vi "solar Unpack.vi"(6 "Timed Out?":bool, 8 "error in (no error)":errorcluster, 9 "DATA in":variant, 10 "MSG in":string, 11 "solar in":refnum<class "solar.lvclass">) -> (0 "error out":errorcluster, 1 "DATA out":variant, 2 "MSG out":string, 3 "solar out":refnum<class "solar.lvclass">)   [LabVIEW 2018, in "solar.lvclass"]
doc: "Handle unpacking custom target messages."
uses:
  solar.lvclass
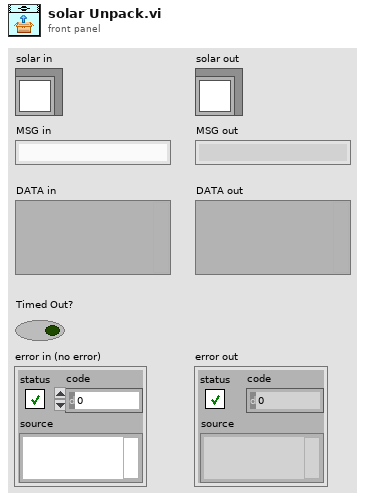
[diagram p1: front panel]
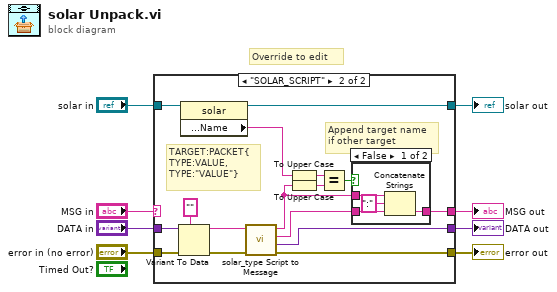
[diagram p0: block diagram]
diagram:
  # "Override to edit"
  n1 = case shown="\"SOLAR_SCRIPT\"" "MSG in" {
    selector: "MSG in" -> [w11 _]
    tunnel: [w12 w22] -> w8
    tunnel: "error in (no error)" -> [w12 w28]
    tunnel: "DATA in" -> [w10 w27]
    tunnel: [w11 w13] -> w4
    tunnel: [w10 w21] -> w5
    tunnel: [w9 w20] -> w2
    tunnel: "solar in" -> [w9 w23]
    frame Default {
    }
    frame "SOLAR_SCRIPT" {
      # "Append target name\nif other target"
      # "TARGET:PACKET{\nTYPE:VALUE,\nTYPE:\"VALUE\"}"
      n2 = Variant To Data(error in=w28, type="", Variant=w27) -> (data=w24:string, error out=w25:errorcluster)
      n3 = property class="solar"(reference=w23) -> (reference out=w20:refnum<class "solar.lvclass">, "Accessors:This.Name"=w19:string)  [unwired: 1 in, 1 out]
      n4 = call "solar_type Script to Message.vi"("error in (no error)"=w25, "Script String"=w24) -> ("error out"=w22:errorcluster, "Data"=w21:variant, "Packet"=w14:string, "Target"=w15:string)  [unwired: 4 in, 2 out]
      n5 = To Upper Case(1:w19) -> (0:w18:string)
      n6 = To Upper Case(1:w15) -> (0:w17:string)
      n7 = Equal?(x=w18, y=w17) -> (x = y?=w16:bool)
      n8 = case shown="False" w16 {
        tunnel: w15 -> [w32 _]
        tunnel: w14 -> [w31 w33]
        tunnel: [w30 w33] -> w13
        frame False {
          n9 = Concatenate Strings(w32, ":" ("string"), w31) -> (w30:string)
        }
        frame True {
        }
      }
    }
  }
  "error out" <- w8
  "solar out" <- w2
  "MSG out" <- w4
  "DATA out" <- w5
